vi "Neocera21 Get Controls.vi"(8 "error in (no error)":errorcluster, 10 "Control Panel Data":T1={"Channels to measure"=[1.0], "Record heater"=FALSE, "Set point"=0.0, "Set Heater Range"=enum."Off", "Control"=FALSE, "Approach"=enum."Instant", "Ramp rate, K/min"=1.0, "Control Channel"=1, "P"=0.0, "I"=0.0, "D"=0.0, "Suspend heater"=FALSE}, 11 "VISA resource name":refnum<visa-resource-name>) -> (0 "error out":errorcluster, 2 "Control Panel Data Out":T1={"Channels to measure"=[1.0], "Record heater"=FALSE, "Set point"=0.0, "Set Heater Range"=enum."Off", "Control"=FALSE, "Approach"=enum."Instant", "Ramp rate, K/min"=1.0, "Control Channel"=1, "P"=0.0, "I"=0.0, "D"=0.0, "Suspend heater"=FALSE}, 3 "VISA Resource Name Out":refnum<visa-resource-name>)   [LabVIEW 2015]
uses:
  Neocera Front Panel Data.ctl
  Neocera Heater Ranges.ctl
  Neocera Set Point Aproach.ctl
  GPIB/VISA  Send Receive.vi
panel:
  out "data string out":string
  out "data string":string
  # "Temperature Monitor"
  # "Temperature Control"
  # "Temperature Monitor"
  # "Temperature Control"
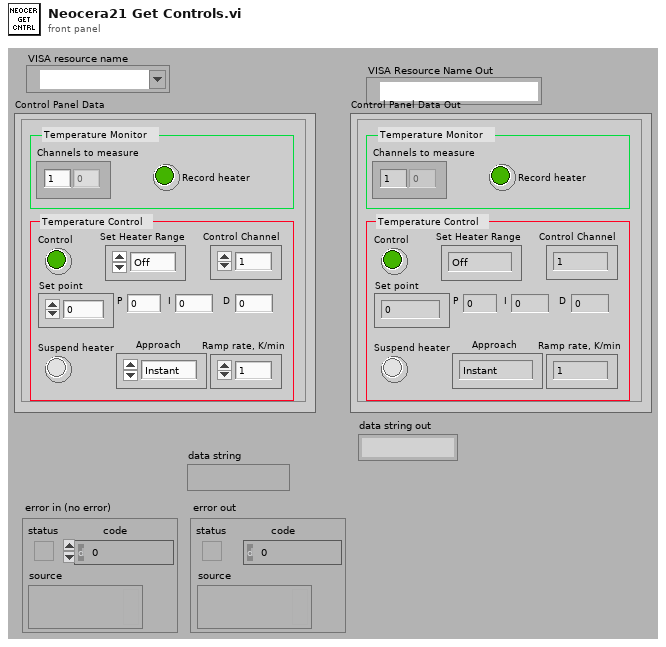
[diagram p1: front panel]
types:
  T1 = typedef "Neocera Front Panel Data.ctl" = cluster{"Channels to measure":dbl[], "Record heater":bool, "Set point":dbl, "Set Heater Range":T2, "Control":bool, "Approach":T3, "Ramp rate, K/min":dbl, "Control Channel":i16, "P":dbl, "I":dbl, "D":dbl, "Suspend heater":bool}
  T2 = typedef "Neocera Heater Ranges.ctl" = enum16{"Off", "0.05W", "0.5W", "5W", "50W"}
  T3 = typedef "Neocera Set Point Aproach.ctl" = enum16{"Instant", "Ramp"}
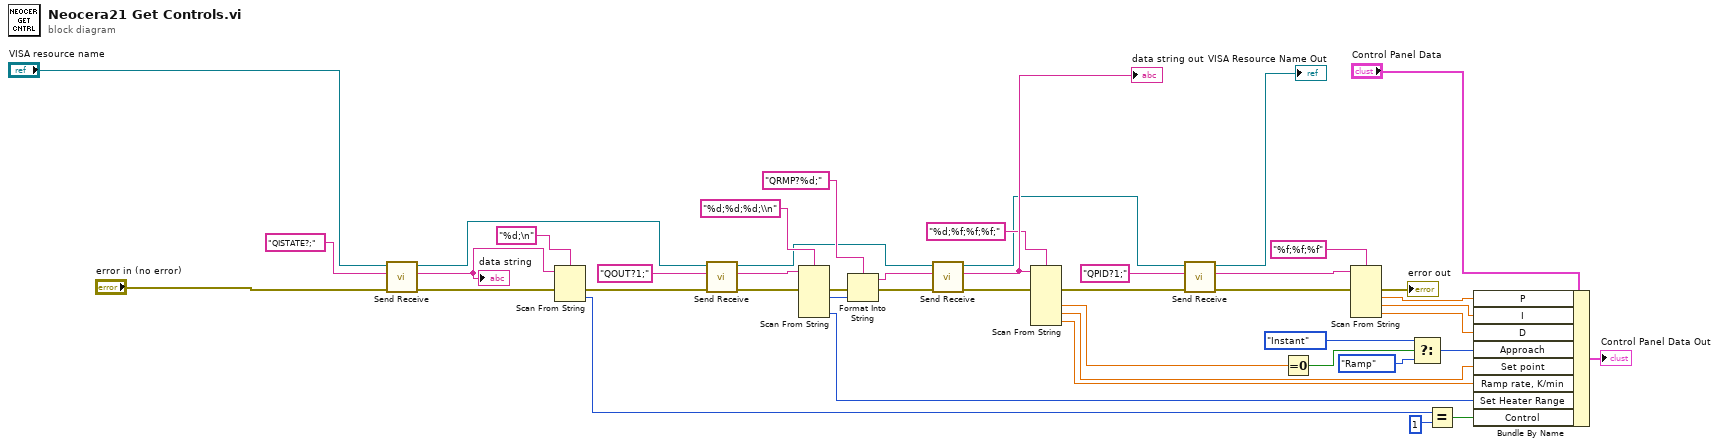
[diagram p0: block diagram]
diagram:
  n1 = call-poly "Send Receive.vi"("error in (no error)"="error in (no error)", "data string in"="QISTATE?;" ("data string"), "VISA Resource Name"="VISA resource name") -> ("error out"=w42:errorcluster, "data string out"=w35:string, "VISA Resource Name Out"=w24:refnum<visa-resource-name>)  [unwired: 6 in]
  "data string" <- w35
  n2 = Scan From String(format string="%d;\n", input string=w35, error in=w42) -> (error out=w29:errorcluster, output 1=w40:i32)  [unwired: 2 in, 2 out]
  n3 = call-poly "Send Receive.vi"("error in (no error)"=w29, "data string in"="QOUT?1;", "VISA Resource Name"=w24) -> ("error out"=w28:errorcluster, "data string out"=w26:string, "VISA Resource Name Out"=w25:refnum<visa-resource-name>)  [unwired: 6 in]
  n4 = Scan From String(format string="%d;%d;%d;\\n", input string=w26, error in=w28) -> (error out=w27:errorcluster, output 1=w6:i32, output 3=w21:i32)  [unwired: 5 in, 2 out]
  n5 = Format Into String(format string="QRMP?%d;", error in=w27, w6) -> (resulting string=w32:string, error out=w33:errorcluster)  [unwired: 1 in]
  n6 = call-poly "Send Receive.vi"("error in (no error)"=w33, "data string in"=w32, "VISA Resource Name"=w25) -> ("error out"=w31:errorcluster, "data string out"=w23:string, "VISA Resource Name Out"=w12:refnum<visa-resource-name>)  [unwired: 6 in]
  "data string out" <- w23
  n7 = Scan From String(format string="%d;%f;%f;%f;", input string=w23, error in=w31) -> (error out=w2:errorcluster, output 2=w18:dbl, output 3=w19:dbl, output 4=w20:dbl)  [unwired: 6 in, 2 out]
  n8 = call-poly "Send Receive.vi"("error in (no error)"=w2, "data string in"="QPID?1;" ("write buffer"), "VISA Resource Name"=w12) -> ("error out"=w8:errorcluster, "data string out"=w9:string, "VISA Resource Name Out"=→"VISA Resource Name Out":refnum<visa-resource-name>)  [unwired: 6 in]
  n9 = Equal To 0?(x=w18) -> (x = 0?=w17:bool)
  n10 = Scan From String(format string="%f;%f;%f", input string=w9, error in=w8) -> (error out=→"error out":errorcluster, output 1=w5:dbl, output 2=w4:dbl, output 3=w3:dbl)  [unwired: 4 in, 2 out]
  n11 = Select(t=Neocera_Set_Point_Aproach."Instant" ("Approach"), s=w17, f=Neocera_Set_Point_Aproach."Ramp" ("Approach")) -> (s? t:f=w14:T3)
  n12 = Equal?(x=w40, y=1) -> (x = y?=w36:bool)
  n13 = Bundle By Name(cluster="Control Panel Data", "P"=w5, "I"=w4, "D"=w3, "Approach"=w14, "Set point"=w19, "Ramp rate, K/min"=w20, "Set Heater Range"=w21, "Control"=w36) -> (→"Control Panel Data Out":T1)
